vi "log.vi"(9 "响应报文":string, 11 "发送报文":string) -> ()   [LabVIEW 2015]
uses:
  <vilib>/Utility/file.llb/Write Delimited Spreadsheet (string).vi
panel:
  in  "URL":string="URL="
  in  "接口耗时":i32
  in  "StartTime":string
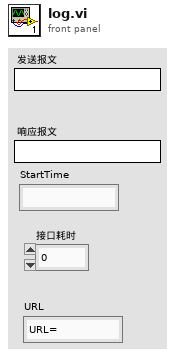
[diagram p1: front panel]
types:
  T1 = enum16{"open", "replace", "create", "open or create", "replace or create", "replace or create with confirmation"}
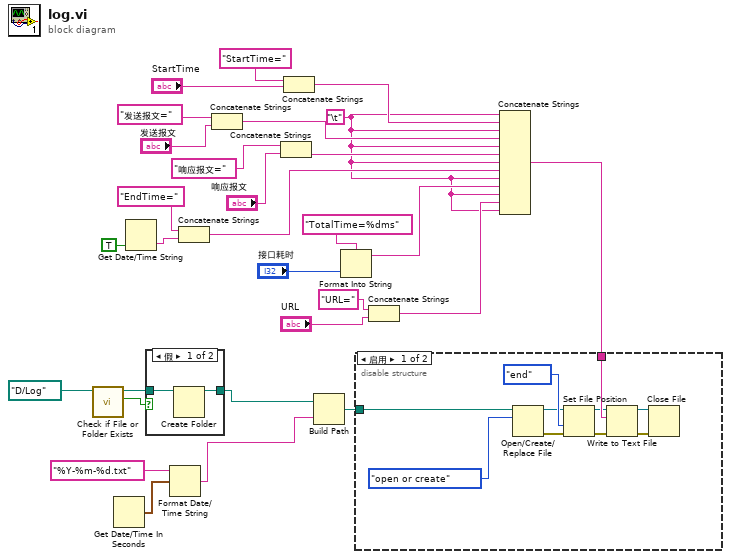
[diagram p0: block diagram]
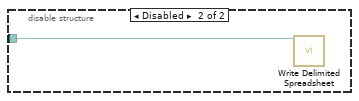
[diagram p2: hidden frame]
diagram:
  w1 = "\t"
  n1 = call <vilib>:"Check if File or Folder Exists.vi"("path"=path "D:/Log" ("路径")) -> ("file or folder exists?"=w25:bool, "dup path"=w26:path)  [unwired: 8 in, 1 out]
  n2 = Get Date/Time In Seconds() -> (seconds since 1Jan1904=w21:timestamp)
  n3 = Get Date/Time String(want seconds? (F)=TRUE ("需要秒？(F)")) -> (time string=w11:string)  [unwired: 2 in, 1 out]
  n4 = case shown="假" w25 {
    tunnel: w26 -> [w31 w32]
    tunnel: [w30 w32] -> w23
    frame False {
      n5 = Create Folder(path (use dialog)=w31) -> (created path=w30:path)  [unwired: 2 in, 2 out]
    }
    frame True {
    }
  }
  n6 = Format Date/Time String(time format string (%c)="%Y-%m-%d.txt" ("时间格式字符串(%c)"), seconds (now)=w21) -> (date/time string=w20:string)  [unwired: 1 in]
  n7 = Concatenate Strings("EndTime=" ("value"), w11) -> (w8:string)
  n8 = Concatenate Strings("发送报文=" ("value"), "发送报文") -> (w14:string)
  n9 = Concatenate Strings("响应报文=" ("value"), "响应报文") -> (w12:string)
  n10 = Concatenate Strings("StartTime=" ("value"), "StartTime") -> (w17:string)
  n11 = Build Path(base path=w23, name or relative path=w20) -> (appended path=w27:path)
  n12 = Format Into String(format string="TotalTime=%dms" ("value"), "接口耗时") -> (resulting string=w5:string)  [unwired: 2 in, 1 out]
  n13 = Concatenate Strings("URL=" ("value"), "URL") -> (w2:string)
  n14 = Concatenate Strings(w1, w17, w1, w14, w1, w12, w1, w8, w1, w5, w1, w2, w1) -> (w29:string)
  n15 = disable-structure shown="启用" {
    disable-tunnel: w29 -> [w42 _]
    disable-tunnel: w27 -> [w33 w43]
    frame Enabled {
      n16 = Open/Create/Replace File(file path (use dialog)=w33, operation (0:open)=T1."open or create" ("操作(0:open)")) -> (refnum out=w37:refnum<file>, error out=w38:errorcluster)  [unwired: 4 in, 1 out]
      n17 = Set File Position(refnum=w37, from (0:start)=enum16{"start", "end", "current"}."end" ("自（0:起始）"), error in=w38) -> (refnum out=w39:refnum<file>, error out=w40:errorcluster)  [unwired: 1 in]
      n18 = Write to Text File(file (use dialog)=w39, text=w42, error in=w40) -> (refnum out=w36:refnum<file>, error out=w35:errorcluster)  [unwired: 1 in, 1 out]
      n19 = Close File(refnum=w36, error in=w35) -> ()  [unwired: 2 out]
    }
    frame Disabled {
      n20 = call-poly <vilib>:"Write Delimited Spreadsheet.vi"("file path (dialog if empty)"=w43) -> ()  [unwired: 13 in, 2 out]
    }
  }
